vi "bank_account_withEvent.vi"() -> ()   [LabVIEW 2022 SP3]
panel:
  in  "Clear":bool
  in  "Exit":bool
  in  "Enter Money":dbl
  in  "Menu":T1(ring)
  out "Balance":dbl
  in  "ENTER":bool
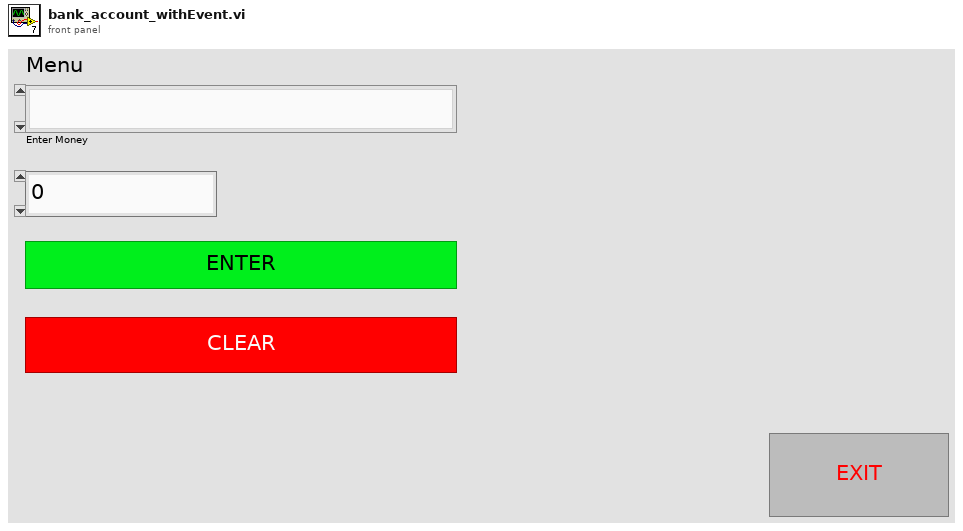
[diagram p1: front panel]
types:
  T1 = enum16{"", "Check Balance", "Cash Withdraw", "Cash Deposit"}
  T2 = enum8{"Enabled", "Disabled", "Disabled and Grayed Out"}
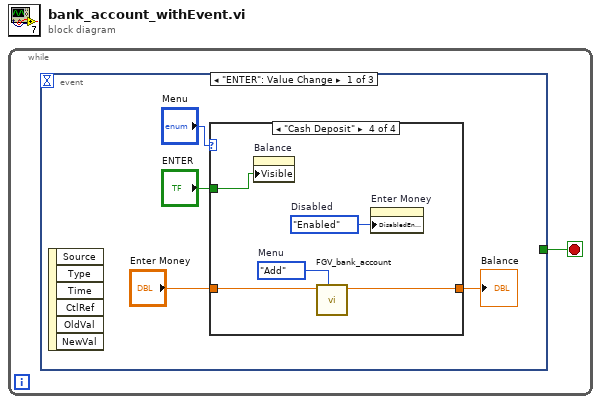
[diagram p0: block diagram]
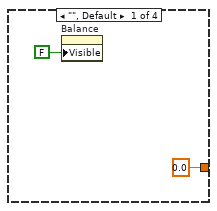
[diagram p2: hidden frame]
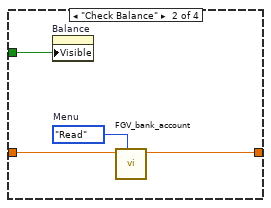
[diagram p3: hidden frame]
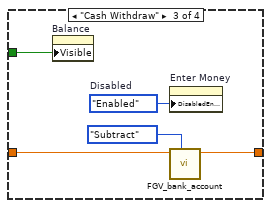
[diagram p4: hidden frame]
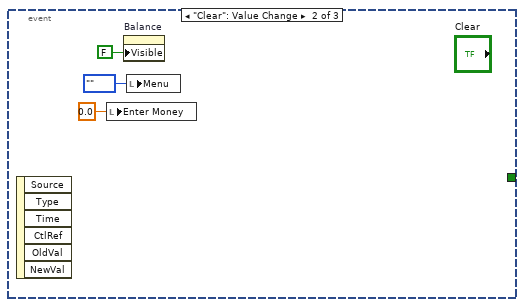
[diagram p5: hidden frame]
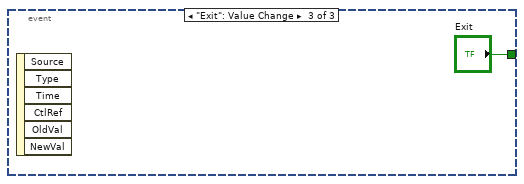
[diagram p6: hidden frame]
diagram:
  n1 = while {
    stop <- w1 stop-if-true
    n2 = event shown="[0] \"ENTER\": Value Change" {
      selector: _ -> [_ _ _]
      dyn-events: _ -> [_ _ _]
      timeout: _ -> [_ _ _]
      tunnel: [_ _ "Exit"] -> w1
      event "ENTER": Value Change {
        n3 = event-data() -> ()  [unwired: 1 in, 6 out]
        n4 = case shown="\"Cash Deposit\"" "Menu" {
          tunnel: "Enter Money" -> [_ w10 w12 w19]
          tunnel: [0.0 w8 w13 w18] -> w3
          tunnel: "ENTER" -> [_ w11 w15 w20]
          frame "", Default {
            n5 = property on="Balance" class="DigNum (strict)"("Visible"=FALSE) -> ()  [unwired: 2 in, 2 out]
          }
          frame "Check Balance" {
            w9 = enum16{"Read", "Subtract", "Add"}."Read"  # Menu
            n6 = property on="Balance" class="DigNum (strict)"("Visible"=w11) -> ()  [unwired: 2 in, 2 out]
            n7 = call "FGV_bank_account.vi"("Menu"=w9, "input"=w10) -> ("Output"=w8:dbl)  [unwired: 8 in, 1 out]
          }
          frame "Cash Withdraw" {
            w16 = T2."Enabled"  # Disabled
            n8 = property on="Balance" class="DigNum (strict)"("Visible"=w15) -> ()  [unwired: 2 in, 2 out]
            n9 = property on="Enter Money" class="DigNum (strict)"("DisabledEnum"=w16) -> ()  [unwired: 2 in, 2 out]
            n10 = call "FGV_bank_account.vi"("Menu"=enum16{"Read", "Subtract", "Add"}."Subtract", "input"=w12) -> ("Output"=w13:dbl)  [unwired: 8 in, 1 out]
          }
          frame "Cash Deposit" {
            w17 = enum16{"Read", "Subtract", "Add"}."Add"  # Menu
            w21 = T2."Enabled"  # Disabled
            n11 = property on="Balance" class="DigNum (strict)"("Visible"=w20) -> ()  [unwired: 2 in, 2 out]
            n12 = call "FGV_bank_account.vi"("Menu"=w17, "input"=w19) -> ("Output"=w18:dbl)  [unwired: 8 in, 1 out]
            n13 = property on="Enter Money" class="DigNum (strict)"("DisabledEnum"=w21) -> ()  [unwired: 2 in, 2 out]
          }
        }
        "Balance" <- w3
      }
      event "Clear": Value Change {
        n14 = event-data() -> ()  [unwired: 1 in, 6 out]
        n15 = local write "Enter Money"(0.0 ("Enter Money")) -> ()
        n16 = property on="Balance" class="DigNum (strict)"("Visible"=FALSE) -> ()  [unwired: 2 in, 2 out]
        n17 = local write "Menu"(T1."" ("Menu")) -> ()
      }
      event "Exit": Value Change {
        n18 = event-data() -> ()  [unwired: 1 in, 6 out]
      }
    }
  }
